vi "ExcelDataToArray.vi"(8 "end cell":string="h8192", 9 "start cell":string="d5", 10 "sheet#":i32=1, 11 "path":path) -> (0 "error out":errorcluster, 3 "data":string[][](array[string]))   [LabVIEW 2012]
panel:
  in  "Excel._Worksheet":refnum<k7>
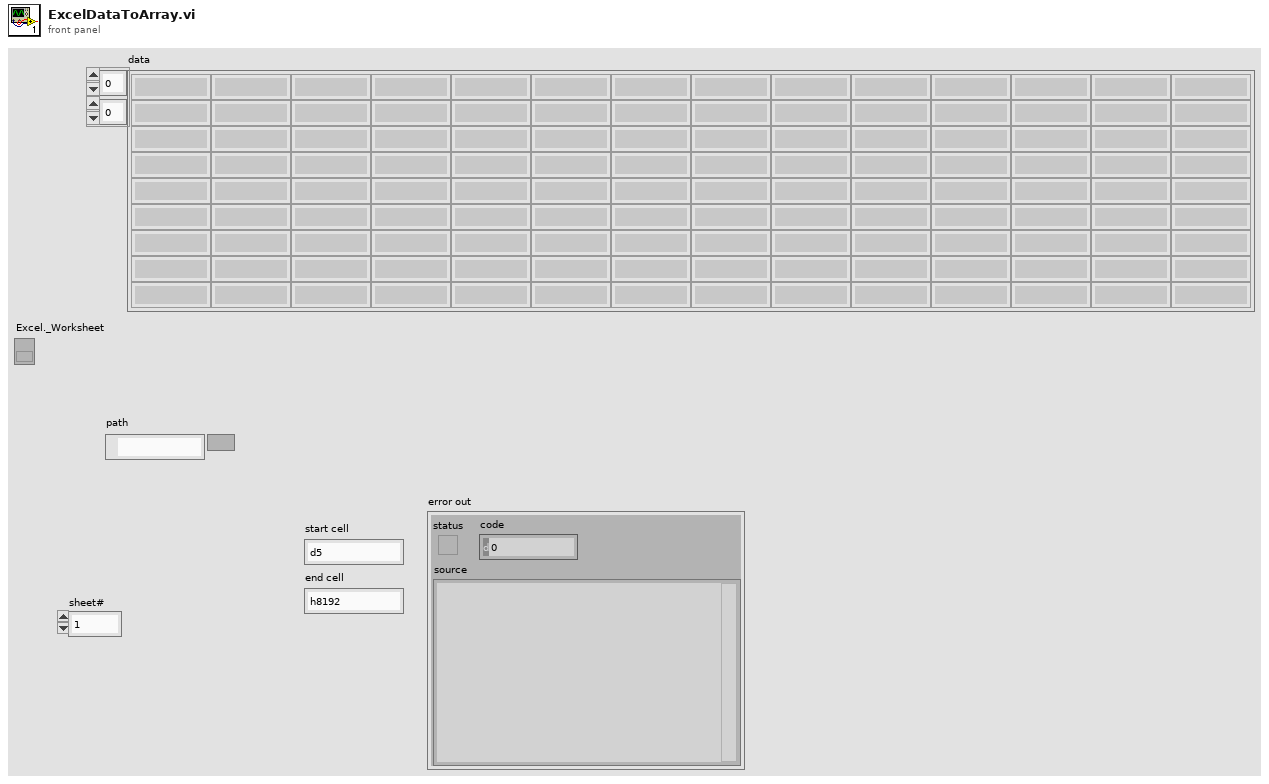
[diagram p1: front panel]
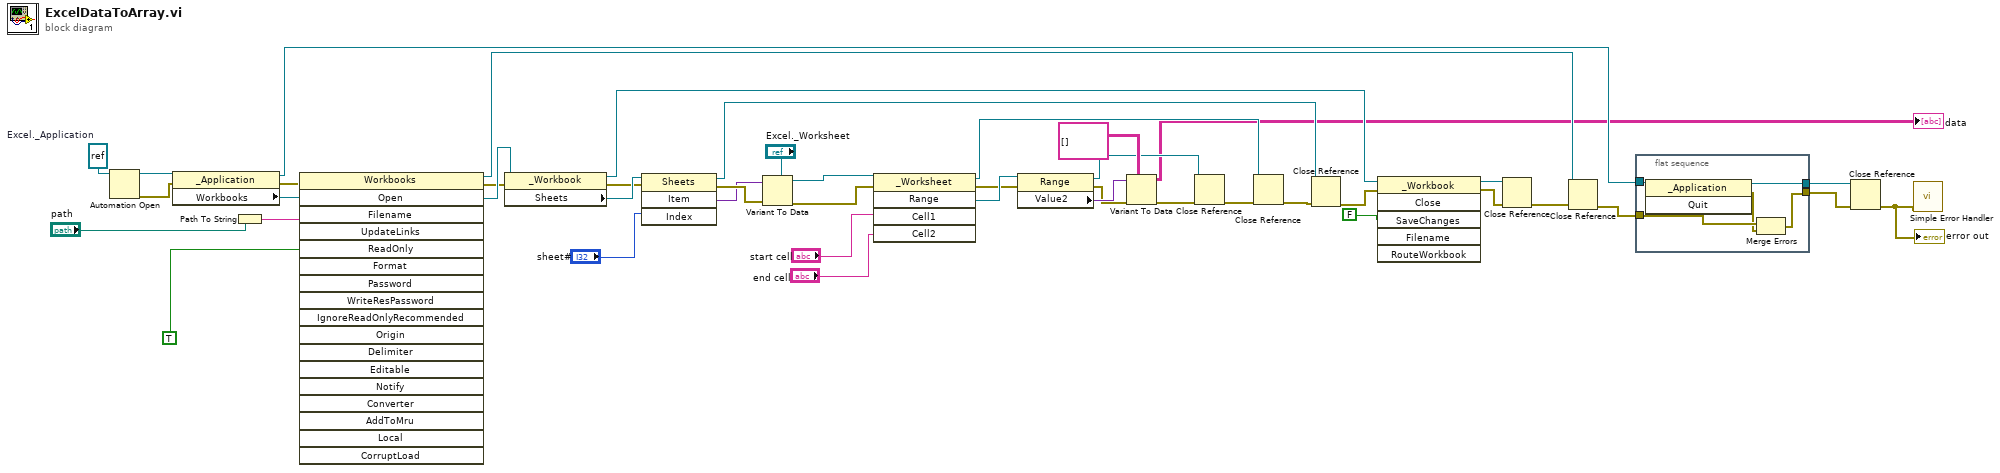
[diagram p0: block diagram]
diagram:
  w12 = refnum<k7> refnum  # Excel._Application
  n1 = Automation Open(Automation Refnum=w12) -> (Automation Refnum=w25:refnum<k7>, error out=w43:errorcluster)  [unwired: 3 in]
  n2 = property class="_Application"(reference=w25, error in=w43) -> (reference out=w15:refnum<k7>, error out=w41:errorcluster, "Workbooks"=w42:refnum<k7>)
  n3 = Path To String(path="path") -> (string=w28:string)
  n4 = invoke class="Workbooks" method="Open"(reference=w42, error in=w41, "Filename"=w28, "ReadOnly"=TRUE) -> (reference out=w3:refnum<k7>, error out=w39:errorcluster, "Open"=w40:refnum<k7>)  [unwired: 14 in, 15 out]
  n5 = property class="_Workbook"(reference=w40, error in=w39) -> (reference out=w22:refnum<k7>, error out=w26:errorcluster, "Sheets"=w38:refnum<k7>)
  n6 = invoke class="Sheets" method="Item"(reference=w38, error in=w26, "Index"="sheet#") -> (reference out=w4:refnum<k7>, error out=w37:errorcluster, "Item"=w36:variant)  [unwired: 1 in, 1 out]
  n7 = Variant To Data(error in=w37, type="Excel._Worksheet", Variant=w36) -> (data=w35:refnum<k7>, error out=w34:errorcluster)
  n8 = invoke class="_Worksheet" method="Range"(reference=w35, error in=w34, "Cell1"="start cell", "Cell2"="end cell") -> (reference out=w6:refnum<k7>, error out=w32:errorcluster, "Range"=w33:refnum<k7>)  [unwired: 1 in, 2 out]
  n9 = property class="Range"(reference=w33, error in=w32) -> (reference out=w5:refnum<k7>, error out=w30:errorcluster, "Value2"=w31:variant)
  n10 = Variant To Data(error in=w30, type=string[][] [], Variant=w31) -> (data=→"data":string[][], error out=w29:errorcluster)
  n11 = Close Reference(reference=w5, error in (no error)=w29) -> (error out=w24:errorcluster)
  n12 = Close Reference(reference=w6, error in (no error)=w24) -> (error out=w23:errorcluster)
  n13 = Close Reference(reference=w4, error in (no error)=w23) -> (error out=w21:errorcluster)
  n14 = invoke class="_Workbook" method="Close"(reference=w22, error in=w21, "SaveChanges"=FALSE) -> (reference out=w19:refnum<k7>, error out=w20:errorcluster)  [unwired: 3 in, 4 out]
  n15 = Close Reference(reference=w19, error in (no error)=w20) -> (error out=w18:errorcluster)
  n16 = Close Reference(reference=w3, error in (no error)=w18) -> (error out=w17:errorcluster)
  n17 = flat-sequence {
    tunnel: w17 -> [w47]
    tunnel: [w45] -> w16
    tunnel: w15 -> [w49]
    tunnel: [w48] -> w14
    frame #0 {
      n18 = invoke class="_Application" method="Quit"(reference=w49) -> (reference out=w48:refnum<k7>, error out=w46:errorcluster)  [unwired: 2 in, 1 out]
      n19 = Merge Errors(w47, w46) -> (w45:errorcluster)
    }
  }
  n20 = Close Reference(reference=w14, error in (no error)=w16) -> (error out=w13:errorcluster)
  "error out" <- w13
  n21 = call <vilib>:"Simple Error Handler.vi"("error in (no error)"=w13) -> ()  [unwired: 4 in, 5 out]
